vi "SCMP - Run Cbk break.vi"(7 "use/init (use)":enum16{"use", "init", "release", "stop"}(ring), 10 "error in (no error)":errorcluster, 11 "user break":bool) -> (2 "error out":errorcluster, 3 "stop loop":bool, 5 "stop ack":bool)   [LabVIEW 2014]
doc: "break subvi na ukoncenie vsetkych paral. sluciek v Data Acq.vi"
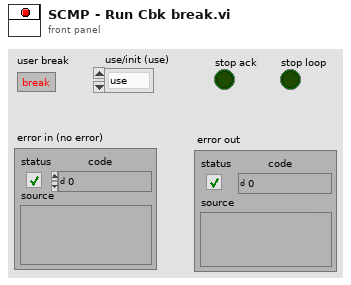
[diagram p1: front panel]
types:
  T1 = typedef "Semaphore RefNum" = refnum<k1>
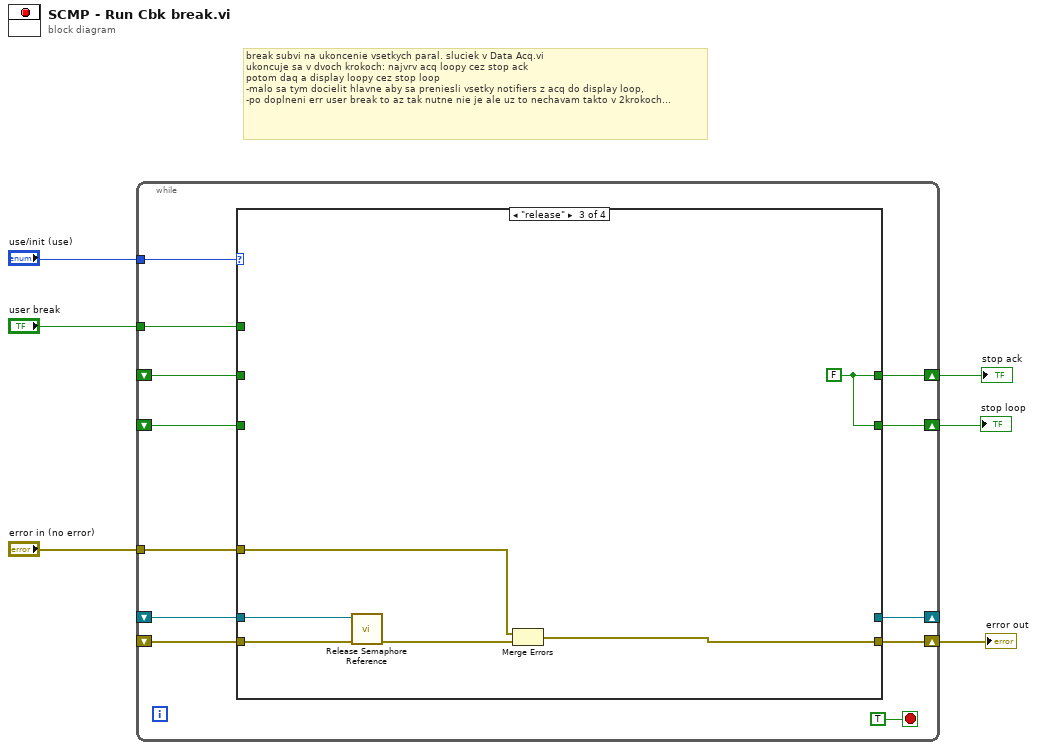
[diagram p0: block diagram]
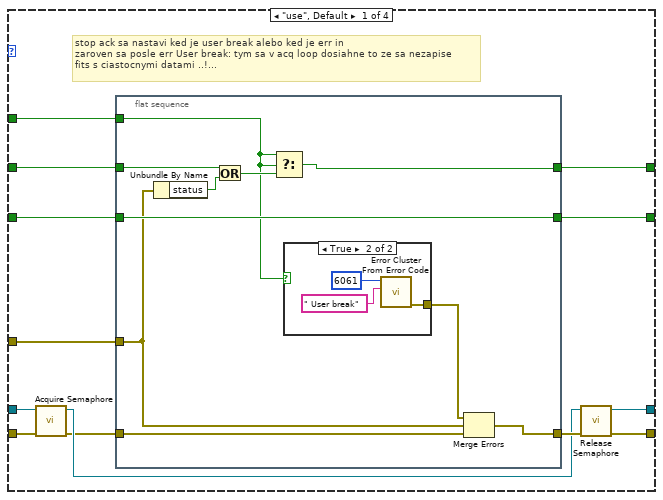
[diagram p2: hidden frame]
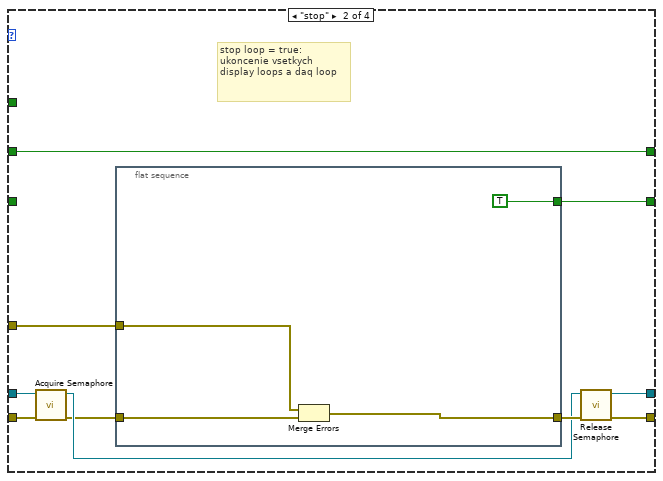
[diagram p4: hidden frame]
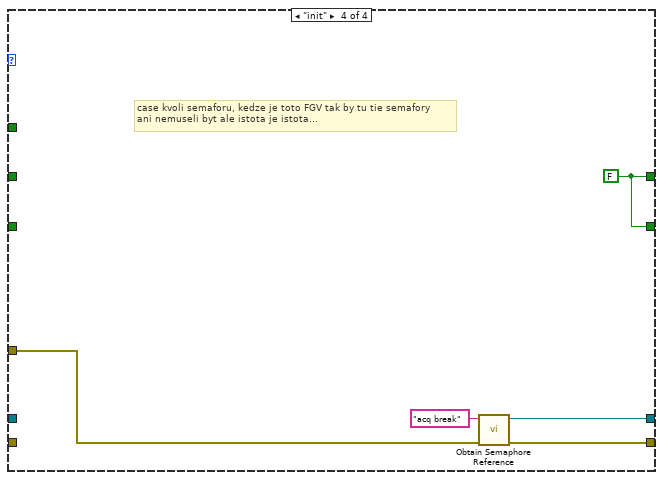
[diagram p5: hidden frame]
diagram:
  # "break subvi na ukoncenie vsetkych paral. sluciek v Data Acq.vi\nukoncuje sa v dvoch krokoch: najvrv acq loopy cez stop ack\npotom daq a display loopy cez stop loop\n-malo sa tym docielit hlavne aby sa preniesli vsetky notifiers z acq do display loop, \n-po doplneni err user break to az tak nutne nie je ale uz to nechavam takto v 2krokoch..."
  n1 = while {
    tunnel: "user break" -> [w17]
    shift-right: [w16] -> w5
    shift-left: _ -> [w15]
    shift-right: [w13] -> _
    shift-left: _ -> [w12]
    tunnel: "use/init (use)" -> [w10]
    shift-right: [w9] -> w2
    shift-left: _ -> [w8]
    shift-right: [w14] -> w4
    shift-left: _ -> [w11]
    tunnel: "error in (no error)" -> [w7]
    stop <- TRUE stop-if-true
    n2 = case shown="\"release\"" w10 {
      tunnel: w17 -> [w31 _ _ _]
      tunnel: [w30 w47 w61 w66] -> w16
      tunnel: w15 -> [w22 w47 _ _]
      tunnel: [w28 w53 w60 w69] -> w14
      tunnel: [w24 w49 _ w68] -> w13
      tunnel: w12 -> [w27 w52 w62 _]
      tunnel: w11 -> [w26 w51 w64 _]
      tunnel: [w20 w46 w61 w66] -> w9
      tunnel: w8 -> [w21 _ _ _]
      tunnel: w7 -> [w19 w45 w59 w65]
      frame "use", Default {
        # "stop ack sa nastavi ked je user break alebo ked je err in\nzaroven sa posle err User break: tym sa v acq loop dosiahne to ze sa nezapise \nfits s ciastocnymi datami ..!..."
        n3 = call <vilib>:"Acquire Semaphore.vi"("error in (no error)"=w26, "semaphore"=w27) -> ("error out"=w23:errorcluster, "semaphore out"=w25:T1)  [unwired: 3 in, 1 out]
        n4 = flat-sequence {
          tunnel: w31 -> [w35]
          tunnel: [w41] -> w30
          tunnel: w23 -> [w36]
          tunnel: [w34] -> w29
          tunnel: w22 -> [w39]
          tunnel: w21 -> [w37]
          tunnel: [w37] -> w20
          tunnel: w19 -> [w32]
          frame #0 {
            n5 = Unbundle By Name(w32) -> ("status"=w38:bool)
            n6 = Or(x=w39, y=w38) -> (x .or. y?=w40:bool)
            n7 = Select(t=w35, s=w35, f=w40) -> (s? t:f=w41:bool)
            n8 = case shown="True" w35 {
              tunnel: [_ w42] -> w33
              frame False {
              }
              frame True {
                n9 = call <vilib>:"Error Cluster From Error Code.vi"("error message (\"\")"=" User break" ("error message (\"\")"), "error code (0)"=6061) -> ("error out"=w42:errorcluster)  [unwired: 7 in]
              }
            }
            n10 = Merge Errors(w33, w32, w36) -> (w34:errorcluster)
          }
        }
        n11 = call <vilib>:"Release Semaphore.vi"("error in (no error)"=w29, "semaphore"=w25) -> ("error out"=w28:errorcluster, "semaphore out"=w24:T1)  [unwired: 4 in]
      }
      frame "stop" {
        # "stop loop = true:\nukoncenie vsetkych display loops a daq loop"
        n12 = call <vilib>:"Acquire Semaphore.vi"("error in (no error)"=w51, "semaphore"=w52) -> ("error out"=w48:errorcluster, "semaphore out"=w50:T1)  [unwired: 3 in, 1 out]
        n13 = flat-sequence {
          tunnel: w48 -> [w58]
          tunnel: [w56] -> w54
          tunnel: [TRUE ("break in")] -> w46
          tunnel: w45 -> [w55]
          frame #0 {
            n14 = Merge Errors(w55, w58) -> (w56:errorcluster)
          }
        }
        n15 = call <vilib>:"Release Semaphore.vi"("error in (no error)"=w54, "semaphore"=w50) -> ("error out"=w53:errorcluster, "semaphore out"=w49:T1)  [unwired: 4 in]
      }
      frame "release" {
        w61 = FALSE ("break in")
        n16 = call <vilib>:"Release Semaphore Reference.vi"("error in (no error)"=w64, "semaphore"=w62) -> ("error out"=w63:errorcluster)  [unwired: 8 in, 1 out]
        n17 = Merge Errors(w59, w63) -> (w60:errorcluster)
      }
      frame "init" {
        w66 = FALSE ("break in")
        # "case kvoli semaforu, kedze je toto FGV tak by tu tie semafory\nani nemuseli byt ale istota je istota..."
        n18 = call <vilib>:"Obtain Semaphore Reference.vi"("error in (no error)"=w65, "name (unnamed)"="acq break") -> ("error out"=w69:errorcluster, "semaphore"=w68:T1)  [unwired: 3 in, 1 out]
      }
    }
  }
  "stop ack" <- w5
  "error out" <- w4
  "stop loop" <- w2
